vi "DCMotorControl_v1.vi"() -> ()   [LabVIEW 2019]
uses:
  <vilib>/myRIO/Common/Instrument Driver Framework/myRIO v1.0/Encoder/typedefs/Encoder Signal Mode.ctl
  <vilib>/myRIO/Instrument Drivers/Onboard IO/Encoder/typedefs/Encoder Reference.ctl
  <vilib>/myRIO/Common/Instrument Driver Framework/Utilities/typedefs/myRIO Generic Hardware Reference.ctl
  <vilib>/myRIO/Common/Instrument Driver Framework/Utilities/typedefs/Hardware Version Enum.ctl
  <vilib>/myRIO/Common/Instrument Driver Framework/Utilities/typedefs/myRIO v1.0 Reference.ctl
  <vilib>/myRIO/Common/Instrument Driver Framework/Utilities/typedefs/Generic FPGA Reference.ctl
  <vilib>/myRIO/Common/Instrument Driver Framework/myRIO v1.0/Encoder/typedefs/Encoder Channels Enum.ctl
  <vilib>/myRIO/Common/Instrument Driver Framework/myRIO v1.0/Encoder/typedefs/Encoder Configuration v1.0.ctl
  <vilib>/userDefined/High Color/nirio_resource_hc.ctl
  <vilib>/Platform/TimedLoop/XDataNode/timing_clust.ctl
  <vilib>/Platform/TimedLoop/XDataNode/nitl_modes.ctl
  <vilib>/Platform/TimedLoop/XDataNode/wakeup.ctl
  <vilib>/myRIO/Instrument Drivers/Onboard IO/DIO/typedefs/DIO Reference.ctl
  <vilib>/myRIO/Common/Instrument Driver Framework/myRIO v1.0/DIO/typedefs/DIO Channels List.ctl
  <vilib>/myRIO/Common/Instrument Driver Framework/myRIO v1.0/DIO/typedefs/DIO Channels Enum.ctl
  <vilib>/myRIO/Instrument Drivers/Onboard IO/PWM/typedefs/PWM Reference.ctl
  <vilib>/myRIO/Common/Instrument Driver Framework/myRIO v1.0/PWM/typedefs/PWM Channels Enum.ctl
  <vilib>/myRIO/Instrument Drivers/Onboard IO/PWM/typedefs/PWM Configuration.ctl
  <vilib>/myRIO/Common/Instrument Driver Framework/Utilities/vis/Is FPGA Ref Available.vi
  <vilib>/myRIO/Common/Instrument Driver Framework/myRIO v1.0/Encoder/vis/myRIO v1.1 Open Encoder.vi
  <vilib>/myRIO/Instrument Drivers/Onboard IO/Encoder/vis/Read.vi
  <vilib>/myRIO/Common/Instrument Driver Framework/myRIO v1.0/DIO/vis/myRIO v1.1 Open DIO.vi
  <vilib>/myRIO/Instrument Drivers/Onboard IO/DIO/vis/Write.vi
  <vilib>/myRIO/Common/Instrument Driver Framework/myRIO v1.0/PWM/vis/myRIO v1.1 Open PWM.vi
  <vilib>/myRIO/Instrument Drivers/Onboard IO/PWM/vis/Set Duty Cycle and Frequency.vi
  <vilib>/myRIO/Common/Instrument Driver Framework/Utilities/vis/Validate Channels.vi
  <vilib>/myRIO/Common/Instrument Driver Framework/myRIO v1.0/Encoder/vis/myRIO v1.0 Reserve Encoder.vi
  <vilib>/myRIO/Common/Instrument Driver Framework/myRIO v1.0/DIO/vis/myRIO v1.0 Reserve DIO.vi
  <vilib>/myRIO/Common/Instrument Driver Framework/myRIO v1.0/PWM/vis/myRIO v1.0 Reserve PWM.vi
  <vilib>/myRIO/Common/Instrument Driver Framework/myRIO v1.0/Encoder/vis/myRIO v1.0 Build MUX Configuration Encoder.vi
  <vilib>/myRIO/Common/Instrument Driver Framework/myRIO v1.0/Resource Manager/vis/myRIO v1.0 Reserve Channel List.vi
  <vilib>/myRIO/Common/Instrument Driver Framework/myRIO v1.0/DIO/vis/myRIO v1.0 Build MUX Configuration DIO.vi
  <vilib>/myRIO/Common/Instrument Driver Framework/myRIO v1.0/PWM/vis/myRIO v1.0 Build MUX Configuration PWM.vi
  <vilib>/myRIO/Common/Instrument Driver Framework/myRIO v1.0/Resource Manager/vis/myRIO v1.0 Create Configuration List.vi
  <vilib>/myRIO/Common/Instrument Driver Framework/myRIO v1.0/Resource Manager/vis/myRIO v1.0 Reserve Channel.vi
  <vilib>/myRIO/Common/Instrument Driver Framework/myRIO v1.0/Resource Manager/vis/myRIO v1.0 Unreserve Channel.vi
  <vilib>/myRIO/Common/Instrument Driver Framework/myRIO v1.0/Resource Manager/vis/myRIO v1.0 Build Mutex Name.vi
  <vilib>/Utility/VariantDataType/GetNumericInfo.vi
  <vilib>/Utility/error.llb/Error Cluster From Error Code.vi
  <vilib>/myRIO/Common/Instrument Driver Framework/myRIO v1.0/myRIO v1.1 Open.vi
  <vilib>/myRIO/Common/Instrument Driver Framework/Utilities/vis/IO Manager.vi
  <vilib>/myRIO/Common/Instrument Driver Framework/Utilities/vis/Configuration Manager.vi
  <vilib>/myRIO/Common/Instrument Driver Framework/myRIO v1.0/Resource Manager/vis/myRIO v1.0 Configure IO.vi
  <vilib>/myRIO/Common/Instrument Driver Framework/myRIO v1.0/myRIO v1.0 Close.vi
  <vilib>/myRIO/Common/Instrument Driver Framework/myRIO v1.0/Encoder/vis/myRIO v1.0 Configure Encoder.vi
  <vilib>/myRIO/Common/Instrument Driver Framework/myRIO v1.0/Encoder/vis/myRIO v1.0 Read Encoder.vi
  <vilib>/myRIO/Common/Instrument Driver Framework/myRIO v1.0/DIO/vis/myRIO v1.0 Write DIO.vi
  <vilib>/myRIO/Common/Instrument Driver Framework/myRIO v1.0/PWM/vis/myRIO v1.0 Write PWM.vi
  <vilib>/Utility/file.llb/Write Delimited Spreadsheet (DBL).vi
  <vilib>/Instr/_visa.llb/VISA Configure Serial Port (Instr).vi
  <vilib>/myRIO/Express VI/Onboard IO/Encoder/Encoder Express VI.xnode
  <vilib>/myRIO/Instrument Drivers/Onboard IO/Encoder/vis/myRIO Encoder Open.xnode
  <vilib>/myRIO/Common/Instrument Driver Framework/myRIO v1.0/Encoder/typedefs/Encoder Count Direction Enum.ctl
  <vilib>/platform/TimedLoop/XDataNode/XDataNode.xnode
  <vilib>/myRIO/Express VI/Onboard IO/DO/DO Express VI.xnode
  <vilib>/myRIO/Instrument Drivers/Onboard IO/DIO/vis/myRIO DIO Open.xnode
  <vilib>/myRIO/Express VI/Onboard IO/PWM/PWM Express VI.xnode
  <vilib>/myRIO/Instrument Drivers/Onboard IO/PWM/vis/myRIO PWM Open.xnode
  <vilib>/myRIO/Instrument Drivers/Onboard IO/PWM/PWM.lvlib
  <vilib>/myRIO/Instrument Drivers/Onboard IO/Encoder/Encoder.lvlib
  <vilib>/Platform/TimedLoop/XDataNode/XDNodeRunTimeDep.lvlib
  <vilib>/myRIO/Instrument Drivers/Onboard IO/DIO/DIO.lvlib
panel:
  in  "stop 2":bool
  in  "VISA resource name 2":refnum<visa-resource-name>
  in  "Baud rate 2":dbl=500000.0
  out "error out 2":errorcluster
  out "read buffer":string
  out "resulting string":string
  in  "Numeric":dbl
  in  "file path (dialog if empty)":path
  in  "format (%.3f)":string="%.3f"
  out "velocity diff (deg/s)":dbl(graph)
  out "angle diff (deg)":dbl(graph)
  out "Duty cycle":dbl(graph)
  out "Time":dbl
  out "Angle_velocity(deg/s)":cluster{"set point":dbl, dbl}(graph)
  out "Angle_velocity(deg/s) Graph":dbl[][](graph)
  out "Angle(deg) Gragh":dbl[][](graph)
  out "Angle(deg)":cluster{dbl, dbl}(graph)
  out "Duty":dbl
  in  "stop":bool
  in  "Frequency [Hz]":dbl=1000.0
  in  "Gain 2":T1={"P Gain"=0.5, "I Gain"=0.0, "D Gain"=0.005}
  out "encoder_position":dbl
  out "Counter Value":i32
  in  "Encoder_Count":dbl=54991.0
  in  "t_shift":dbl=0.000125
  in  "T_ratio":dbl=10.0
  in  "buffer ratio":dbl=0.3
  in  "first or second tripod":bool
  in  "data of 5th order formula\nts,tair,a1-a6":dbl[](array[numeric])
  in  "Loop Period":i64=5
  # "RC Servo Motor"
  # "v = 1; a = 15"
  # "v = 1.25; a = 15"
  # "v = 1.5; a = 15"
  # "0.184067181524967\n0.263820978418769\n256152.551336786\n-30272.30000274\n-9876.03760433421\n-1096.38594197941\n885.91817900106\n-44.6781799901984"
  # "0.215241998794118\n0.254514142390288\n4771.41078363533\n62185.8763006578\n-22508.5336527453\n390.805502041188\n686.695311017595\n-40.4128145310291"
  # "0.163616269216122\n0.27489641502463\n771965.39318528\n-201617.027694185\n8828.08396944145\n-2683.04589908678\n1085.57303422127\n-48.5860395324432"
  # "DC Motor"
  # "v = 1.75; a = 15"
  # "v = 2; a = 15"
  # "v = 2.25; a = 15"
  # "0.148651048423414\n0.288542414074344\n1776973.44893281\n-511591.467559457\n38775.9830765103\n-4576.94506688942\n1289.39828252671\n-52.3115561007577"
  # "0.136976185169818\n0.304016701267508\n3461279.85083822\n-993110.73746345\n80544.6579529191\n-6699.48295844177\n1494.82265451498\n-55.8934424469099"
  # "0.134381902205816\n0.369022171779704\n3272804.8365432\n-899365.569589567\n71225.2463409934\n-7039.10791102172\n1512.66147498591\n-59.3408899720725"
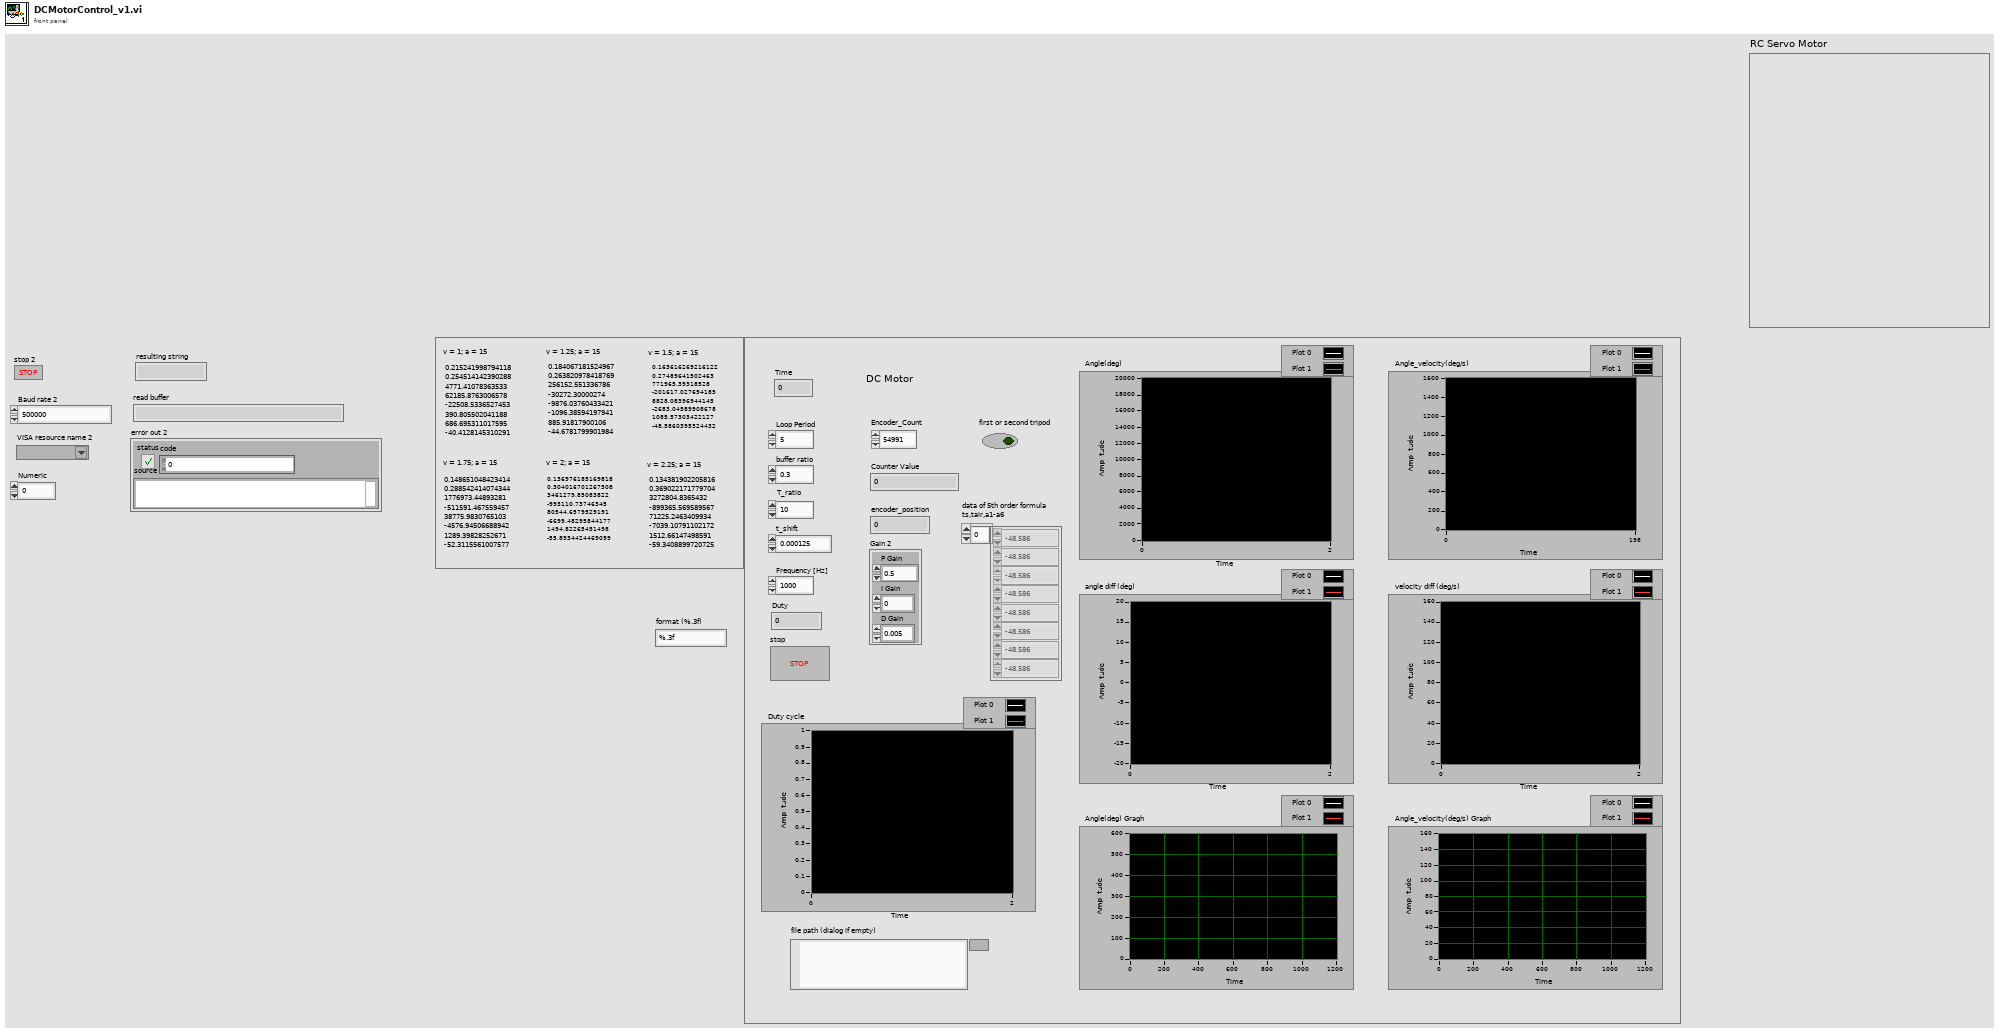
[diagram p1: front panel]
types:
  T1 = cluster{"P Gain":dbl, "I Gain":dbl, "D Gain":dbl}
  T2 = typedef "Encoder.lvlib/Encoder Reference.ctl" = cluster{"myRIO Reference":T3, "Encoder Channels Enum":T7}
  T3 = typedef "myRIO Generic Hardware Reference.ctl" = cluster{"myRIO Model":T4, "myRIO Hardware Reference":T5}
  T4 = typedef "Hardware Version Enum.ctl" = enum16{"Unknown", "myRIO-1900", "myRIO-1950", "roboRIO", "NI ELVIS RIO CM", "ELVIS III"}
  T5 = typedef "myRIO v1.0 Reference.ctl" = cluster{"Generic FPGA Reference":T6, "Allow multiple opens":bool}
  T6 = typedef "Generic FPGA Reference.ctl" = refnum<k20>
  T7 = typedef "Encoder Channels Enum.ctl" = enum16{"Not Connected", "C/ENC0", "C/ENC1", "A/ENC", "A/ENC0", "A/ENC1", "A/ENC2", "A/ENC3", "A/ENC4", "A/ENC5", "A/ENC6", "A/ENC7", "A/ENC8", "A/ENC9", "B/ENC", "B/ENC0", "B/ENC1", "B/ENC2", "B/ENC3", "B/ENC4", "B/ENC5", "B/ENC6", "B/ENC7", "B/ENC8", "B/ENC9", "DIO/ENC0", "DIO/ENC1", "DIO/ENC2", "DIO/ENC3", "DIO/ENC4"}
  T8 = typedef "Encoder Signal Mode.ctl" = enum16{"Quadrature phase signal", "Step and direction signal"}
  T9 = typedef "nirio_resource_hc.ctl" = tag
  T10 = cluster{"set position":dbl, "set position":dbl, "set position":dbl, "set position":dbl, "set position":dbl, "set position":dbl}
  T11 = typedef "DIO.lvlib/DIO Reference.ctl" = cluster{"myRIO Reference":T3, "DIO Channels List":T12}
  T12 = typedef "DIO Channels List.ctl" = T13[]
  T13 = typedef "DIO Channels Enum.ctl" = enum16{"Not Connected", "C/DIO0", "C/DIO1", "C/DIO2", "C/DIO3", "C/DIO4", "C/DIO5", "C/DIO6", "C/DIO7", "A/DIO0", "A/DIO1", "A/DIO2", "A/DIO3", "A/DIO4", "A/DIO5", "A/DIO6", "A/DIO7", "A/DIO8", "A/DIO9", "A/DIO10", "A/DIO11", "A/DIO12", "A/DIO13", "A/DIO14", "A/DIO15", "A/DIO16", "A/DIO17", "A/DIO18", "A/DIO19", "B/DIO0", "B/DIO1", "B/DIO2", "B/DIO3", "B/DIO4", "B/DIO5", "B/DIO6", "B/DIO7", "B/DIO8", "B/DIO9", "B/DIO10", "B/DIO11", "B/DIO12", "B/DIO13", "B/DIO14", "B/DIO15", "B/DIO16", "B/DIO17", "B/DIO18", "B/DIO19", "LED0", "LED1", "LED2", "LED3", "Button0", "DIO/DIO0", "DIO/DIO1", "DIO/DIO2", "DIO/DIO3", "DIO/DIO4", "DIO/DIO5", "DIO/DIO6", "DIO/DIO7", "DIO/DIO8", "DIO/DIO9", "SPI/CS0", "SPI/CS1", "SPI/CS2", "SPI/CS3", "LED RADIO (Green)", "LED RADIO (Red)", "LED COMM (Green)", "LED COMM (Red)", "LED MODE (Green)", "LED MODE (Red)"}
  T14 = typedef "PWM.lvlib/PWM Reference.ctl" = cluster{"myRIO Reference":T3, "PWM Channels Enum":T15, "PWM Configuration":T16}
  T15 = typedef "PWM Channels Enum.ctl" = enum16{"Not Connected", "C/PWM0", "C/PWM1", "A/PWM0", "A/PWM1", "A/PWM2", "A/PWM3", "A/PWM4", "A/PWM5", "A/PWM6", "A/PWM7", "A/PWM8", "A/PWM9", "A/PWM10", "A/PWM11", "A/PWM12", "A/PWM13", "A/PWM14", "A/PWM15", "A/PWM16", "A/PWM17", "A/PWM18", "A/PWM19", "B/PWM0", "B/PWM1", "B/PWM2", "B/PWM3", "B/PWM4", "B/PWM5", "B/PWM6", "B/PWM7", "B/PWM8", "B/PWM9", "B/PWM10", "B/PWM11", "B/PWM12", "B/PWM13", "B/PWM14", "B/PWM15", "B/PWM16", "B/PWM17", "B/PWM18", "B/PWM19", "PWM/PWM0", "PWM/PWM1", "PWM/PWM2", "PWM/PWM3", "PWM/PWM4", "PWM/PWM5", "PWM/PWM6", "PWM/PWM7", "PWM/PWM8", "PWM/PWM9"}
  T16 = typedef "PWM.lvlib/PWM Configuration.ctl" = cluster{"Frequency":dbl, "Duty Cycle":dbl}
  T17 = typedef "XDNodeRunTimeDep.lvlib/timing_clust.ctl" = cluster{"Expected End [f-1]":u64, "Actual End [f-1]":u64, "Finished Late? [f-1]":bool, "Expected End [i-1]":u64, "Actual End [i-1]":u64, "Finished Late? [i-1]":bool, "Expected Start [i]":u64, "Actual Start [i]":u64, "Expected Start [f]":u64, "Actual Start [f]":u64, "Source Name":string, "Structure Name":string, "Period":i64, "Deadline":i64, "Offset":i64, "Start":i64, "Priority":i32, "Timeout":i32, "Mode":T18, "Wakeup Reason":T19, "Error":errorcluster, "Source Type":string, "Secondary Source Type":string, "Global End Time":u64, "Global Start Time":u64, "Frame Duration":u64, "Iteration Duration":u64, "Assigned CPU":i32, "I/O Scan Engine Mode":u32}
  T18 = typedef "XDNodeRunTimeDep.lvlib/nitl_modes.ctl" = enum32{"No Change", "Process missed periods, maintain original phase", "Discard missed periods, maintain original phase", "Process missed periods, ignore original phase", "Discard missed periods, ignore original phase"}
  T19 = typedef "XDNodeRunTimeDep.lvlib/wakeup.ctl" = enum32{"Normal", "Aborted", "Asynchronous wakeup", "Timing source error", "Timed loop error", "Timeout"}
  T20 = cluster{"[0]":dbl, "[1]":dbl, "[2]":dbl, "[3]":dbl, "[4]":dbl, "[5]":dbl}
  T21 = cluster{"set position":i32, "set position":i32, "set position":i32, "set position":i32, "set position":i32, "set position":i32}
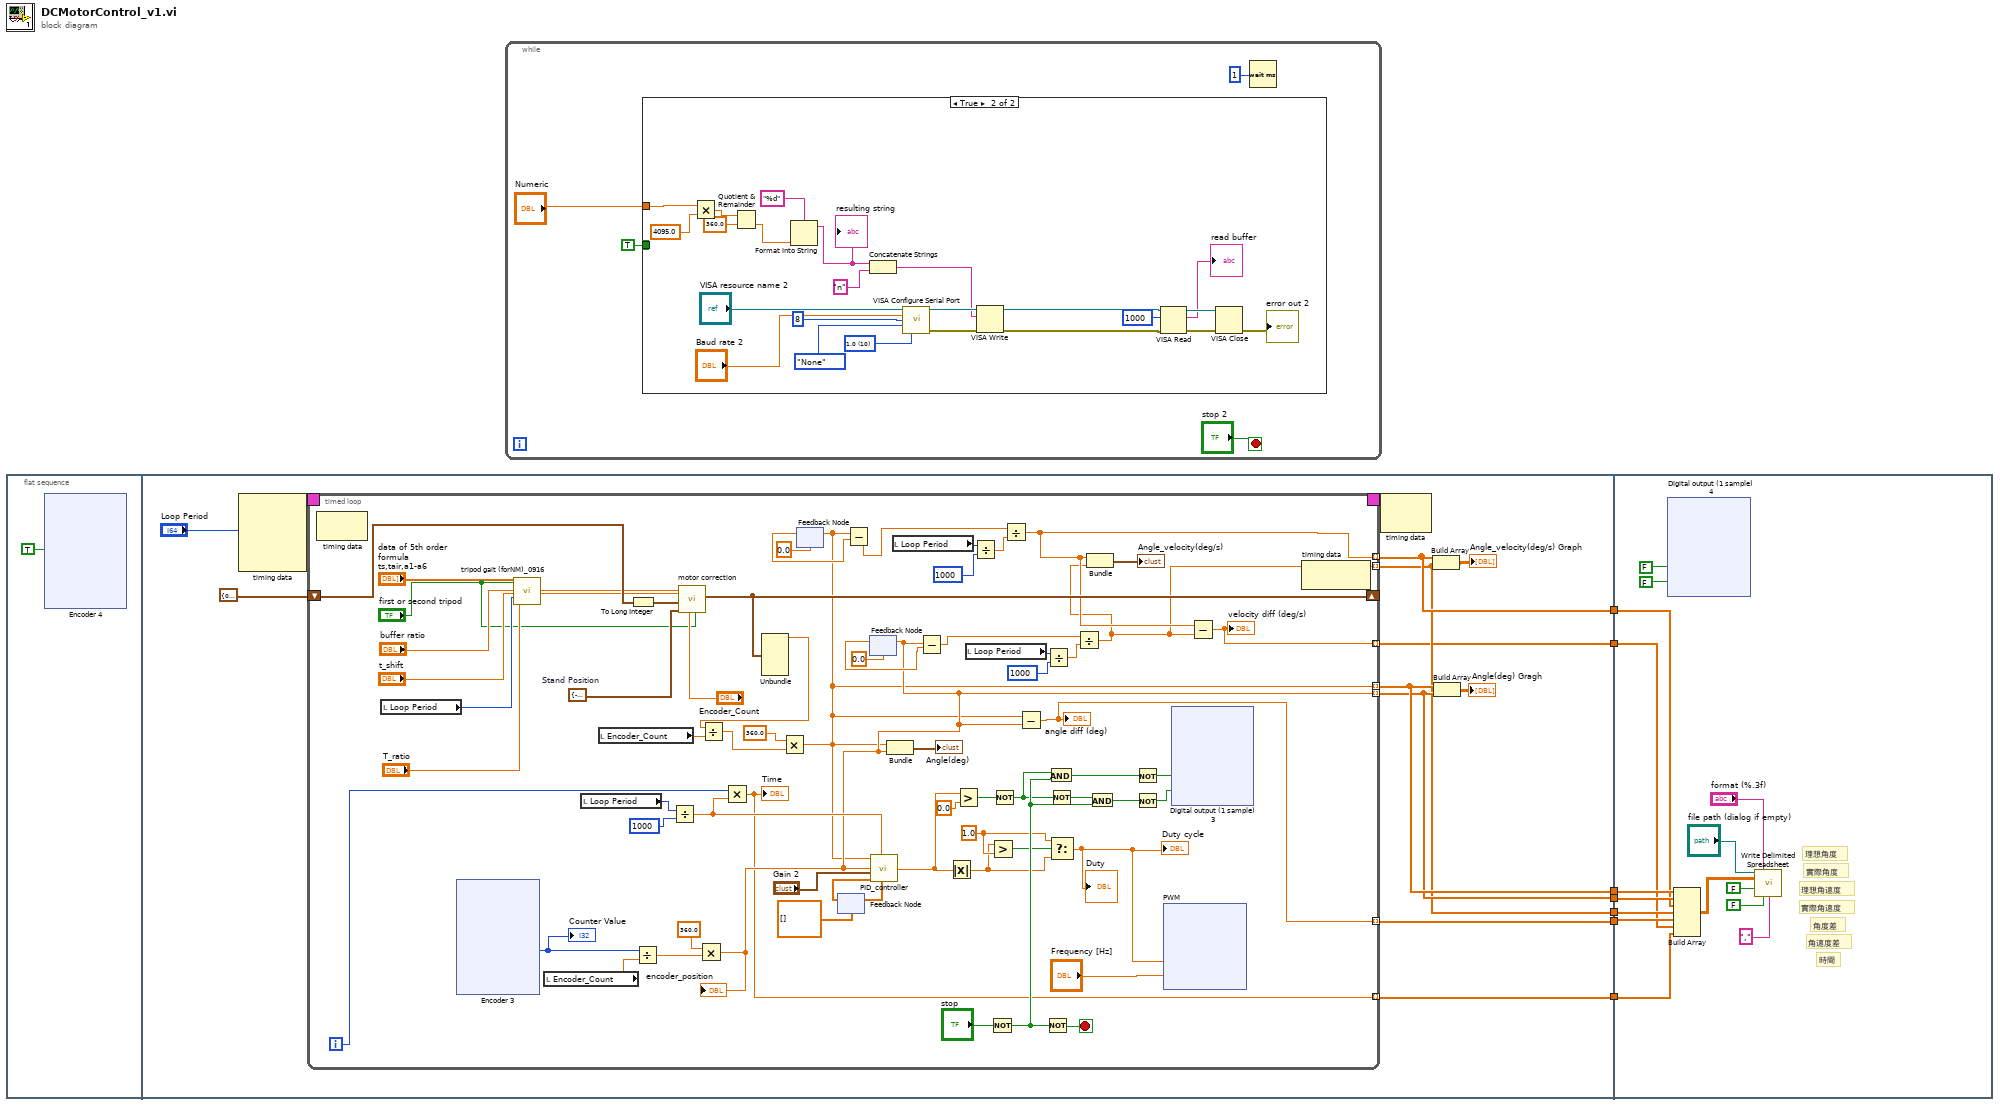
[diagram p0: block diagram]
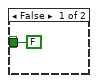
[diagram p2: hidden frame]
diagram:
  n1 = flat-sequence {
    tunnel: [w61] -> w7
    tunnel: [w60] -> w6
    tunnel: [w59] -> w5
    tunnel: [w58] -> w4
    tunnel: [w57] -> w3
    tunnel: [w56] -> w2
    tunnel: [w55] -> w1
    tunnel: w7 -> [w269]
    tunnel: w6 -> [w268]
    tunnel: w5 -> [w267]
    tunnel: w4 -> [w266]
    tunnel: w3 -> [w265]
    tunnel: w2 -> [w264]
    tunnel: w1 -> [w262]
    frame #0 {
      n2 = xnode "Encoder 4"("Reset Counter"=TRUE) -> ()  [unwired: 1 in, 4 out]
    }
    frame #1 {
      n3 = node-c288("Loop Period") -> (w67:T17)  [unwired: 3 in]
      n4 = timed-loop {
        timing: w67 -> [_]
        timing-out: [_] -> w66
        shift-right: [w126] -> _
        shift-left: T10 {"set position"=0.0, "set position"=0.0, "set position"=0.0, "set position"=0.0, "set position"=0.0, "set position"=0.0} ("Setpoint_to_motor") -> [w124]
        tunnel: [w74] -> w60 mode=indexing
        tunnel: [w71] -> w61 mode=indexing
        tunnel: [w72] -> w58 mode=indexing
        tunnel: [w73] -> w59 mode=indexing
        tunnel: [w70] -> w57 mode=indexing
        tunnel: [w69] -> w56 mode=indexing
        tunnel: [w68] -> w55 mode=indexing
        i -> [w82]
        stop <- w103 stop-if-true
        w111 = 1.0 ("y")
        w123 = T20 {"[0]"=-27495.5, "[1]"=-27495.5, "[2]"=-27495.5, "[3]"=-27495.5, "[4]"=-27495.5, "[5]"=-27495.5}  # Stand Position
        n5 = node-c288() -> ()  [unwired: 1 in, 1 out]
        n6 = local read "Loop Period"() -> (w130:i64)
        n7 = xnode "Encoder 3"() -> ("Counter Value"=w76:i32)  [unwired: 2 in, 3 out]
        "Counter Value" <- w76
        n8 = call "tripod gait (forNM)_0916.vi"("data of 5th order formula\nts,tair,a1-a6"="data of 5th order formula\nts,tair,a1-a6", "first or second"="first or second tripod", "buffer ratio"="buffer ratio", "t_shift"="t_shift", "sample time"=w130, "T_ratio"="T_ratio") -> ("Set Point"=w86:dbl, "Set Point 2"=w85:dbl)  [unwired: 4 in, 16 out]
        n9 = local read "Encoder_Count"() -> (w127:dbl)
        n10 = local read "Loop Period"() -> (w94:i64)
        n11 = local read "Encoder_Count"() -> (w92:dbl)
        n12 = To Long Integer(number=w124) -> (32bit integer=w125:T21)
        n13 = Divide(x=w76, y=w127) -> (x/y=w87:dbl)
        n14 = Divide(x=w94, y=i64 1000) -> (x/y=w83:dbl)
        n15 = call "motor correction.vi"("first or second"="first or second tripod", "Encoder_Count"="Encoder_Count", "Stand Position"=w123, "encoder position"=w125, "set position 2"=w85, "set position"=w86) -> ("Setpoint_to_motor"=w126:T10)  [unwired: 4 in, 1 out]
        n16 = Multiply(x=360.0, y=w87) -> (x*y=w74:dbl)
        "encoder_position" <- w74
        n17 = Multiply(x=w82, y=w83) -> (x*y=w68:dbl)
        "Time" <- w68
        n18 = Unbundle(w126) -> ("set position"=w81:dbl)  [unwired: 5 out]
        n19 = Divide(x=w81, y=w92) -> (x/y=w90:dbl)
        n20 = Multiply(x=360.0, y=w90) -> (x*y=w71:dbl)
        n21 = feedback #1(0.0) -> (w98:dbl)
        n22 = feedback-in #1(w71) -> ()
        n23 = feedback #2(dbl[] [] ("state(k)")) -> (w122:dbl[])
        n24 = Subtract(x=w71, y=w98) -> (x-y=w79:dbl)
        n25 = feedback #3(0.0) -> (w78:dbl)
        n26 = feedback-in #3(w74) -> ()
        n27 = call "PID_controller.vi"("Time Period"=w83, "state(k-1)"=w122, "Gain"="Gain 2", "variable"=w74, "set point"=w71) -> ("PID gain"=w104:dbl, "state(k)"=w121:dbl[])
        n28 = feedback-in #2(w121) -> ()
        n29 = Bundle(w71, w74) -> (→"Angle(deg)":cluster{dbl, dbl})  [unwired: 1 in]
        n30 = local read "Loop Period"() -> (w97:i64)
        n31 = Subtract(x=w74, y=w78) -> (x-y=w80:dbl)
        n32 = Absolute Value(x=w104) -> (abs(x)=w110:dbl)
        n33 = Greater?(x=w104, y=0.0) -> (0:w113:bool)
        n34 = local read "Loop Period"() -> (w101:i64)
        n35 = Divide(x=w97, y=i64 1000) -> (x/y=w96:dbl)
        n36 = Not(x="stop") -> (.not. x?=w115:bool)
        n37 = Greater?(x=w110, y=w111) -> (0:w112:bool)
        n38 = Not(x=w113) -> (.not. x?=w109:bool)
        n39 = Divide(x=w79, y=w96) -> (x/y=w73:dbl)
        n40 = Subtract(x=w71, y=w74) -> (x-y=w70:dbl)
        "angle diff (deg)" <- w70
        n41 = Not(x=w115) -> (.not. x?=w103:bool)
        n42 = Divide(x=w101, y=i64 1000) -> (x/y=w99:dbl)
        n43 = And(x=w109, y=w115) -> (x .and. y?=w106:bool)
        n44 = Not(x=w109) -> (.not. x?=w117:bool)
        n45 = Select(t=w111, s=w112, f=w110) -> (s? t:f=w75:dbl)
        "Duty" <- w75
        "Duty cycle" <- w75
        n46 = Divide(x=w80, y=w99) -> (x/y=w72:dbl)
        n47 = Bundle(w73, w72) -> (→"Angle_velocity(deg/s)":cluster{dbl, dbl})  [unwired: 1 in]
        n48 = And(x=w117, y=w115) -> (x .and. y?=w108:bool)
        n49 = Not(x=w106) -> (.not. x?=w105:bool)
        n50 = Not(x=w108) -> (.not. x?=w107:bool)
        n51 = xnode "PWM"("Duty Cycle"=w75, "Frequency [Hz]"="Frequency [Hz]") -> ()  [unwired: 1 in, 1 out]
        n52 = xnode "Digital output (1 sample) 3"("A/DIO0 (Pin 11)"=w105, "A/DIO1 (Pin 13)"=w107) -> ()  [unwired: 1 in, 1 out]
        n53 = Subtract(x=w73, y=w72) -> (x-y=w69:dbl)
        "velocity diff (deg/s)" <- w69
        n54 = node-c288() -> ()  [unwired: 1 in, 1 out]
      }
      n55 = node-c288(w66) -> ()  [unwired: 1 out]
      n56 = Build Array(w59, w58) -> (→"Angle_velocity(deg/s) Graph":dbl[][])
      n57 = Build Array(w61, w60) -> (→"Angle(deg) Gragh":dbl[][])
    }
    frame #2 {
      # "時間"
      # "角速度差"
      # "角度差"
      # "實際角度"
      # "理想角度"
      # "實際角速度"
      # "理想角速度"
      n58 = xnode "Digital output (1 sample) 4"("A/DIO0 (Pin 11)"=FALSE, "A/DIO1 (Pin 13)"=FALSE) -> ()  [unwired: 1 in, 1 out]
      n59 = Build Array(w269, w268, w267, w266, w265, w264, w262) -> (w263:dbl[][])
      n60 = call-poly <vilib>:"Write Delimited Spreadsheet.vi"("file path (dialog if empty)"="file path (dialog if empty)", "format (%.3f)"="format (%.3f)", "2D data"=w263, "append to file? (new file:F)"=FALSE, "transpose? (no:F)"=FALSE, "delimiter (\\t)"="," ("delimiter (\\t)")) -> ()  [unwired: 8 in, 2 out]
    }
  }
  n61 = while {
    stop <- "stop 2" stop-if-true
    n62 = case shown="True" TRUE {
      selector: TRUE -> [_ w314]
      tunnel: "Numeric" -> [_ w322]
      tunnel: [FALSE w314] -> _
      frame False {
      }
      frame True {
        w333 = u16 10 items=["1.0"=10, "1.5"=15, "2.0"=20] ("stop bits (10: 1 bit)")
        n63 = Multiply(x=w322, y=4095.0) -> (x*y=w320:dbl)
        n64 = Quotient & Remainder(x=w320, y=360.0) -> (floor(x/y)=w318:dbl)  [unwired: 1 out]
        n65 = Format Into String(format string="%d", w318) -> (resulting string=w315:string)  [unwired: 2 in, 1 out]
        "resulting string" <- w315
        n66 = Concatenate Strings(w315, "n" ("string")) -> (w325:string)
        n67 = call-poly "VISA Configure Serial Port"("VISA resource name"="VISA resource name 2", "baud rate (9600)"="Baud rate 2", "data bits (8)"=u16 8, "parity (0:none)"=enum16{"None", "Odd", "Even", "Mark", "Space"}."None", "stop bits (10: 1 bit)"=w333) -> ("VISA resource name out"=w332:refnum<visa-resource-name>, "error out"=w331:errorcluster)  [unwired: 9 in]
        n68 = VISA Write(VISA resource name=w332, write buffer=w325, error in (no error)=w331) -> (VISA resource name out=w324:refnum<visa-resource-name>, error out=w323:errorcluster)  [unwired: 1 out]
        n69 = VISA Read(VISA resource name=w324, byte count=u32 1000, error in (no error)=w323) -> (VISA resource name out=w330:refnum<visa-resource-name>, read buffer=→"read buffer":string, error out=w329:errorcluster)  [unwired: 1 out]
        n70 = VISA Close(VISA resource name=w330, error in (no error)=w329) -> (error out=→"error out 2":errorcluster)
      }
    }
    n71 = Wait (ms)(milliseconds to wait=u32 1) -> ()  [unwired: 1 out]
  }
